vi "getExcitation.vi"(8 "error in (no error)":errorcluster, 11 "Inst.AH2500 in":refnum<class "Inst.AH2500.lvclass">) -> (0 "error out":errorcluster, 2 "Excitation (V)":dbl, 3 "Inst.AH2500 out":refnum<class "Inst.AH2500.lvclass">)   [LabVIEW 2019, in "Inst.AH2500.lvclass"]
uses:
  Inst.AH2500.lvclass
  C:/Program Files/National Instruments/LabVIEW 2019/user.lib/LevyLab/Instrument Framework/Instrument/Instrument.lvclass
  Typedefs/Inst.AH2500.Commands--Enum.ctl
  Typedefs/Inst.AH2500.getAll--Cluster.ctl
  991804cd-2d63-4689-a149-8f7b841441b7.vi/c179c0c8-4b72-489b-bcdd-bdfffdae94c9.vi
  991804cd-2d63-4689-a149-8f7b841441b7.vi/c179c0c8-4b72-489b-bcdd-bdfffdae94c9.vi/045b885c-8c33-4e8e-937d-f5afebc728a8.vi
  991804cd-2d63-4689-a149-8f7b841441b7.vi/c179c0c8-4b72-489b-bcdd-bdfffdae94c9.vi/f638782e-dab2-4f71-a606-cfbdff2ea2be.vi
  <vilib>/Utility/Data Type/Get Type Information.vi
  <vilib>/JDP Science/JSONtext/JSON text to Variant.vi
  <vilib>/JDP Science/JSONtext/LVClass Serializer/JSONtext LVClass Serializer.lvclass
  <userlib>/LevyLab/Instrument Framework/Instrument/Instrument.lvclass
  f3cb8313-5d80-4493-8332-6bf410390232.vi
  C:/Program Files/National Instruments/LabVIEW 2019/user.lib/LevyLab/Instrument Framework/Instrument Types/CBridge/Instrument.CBridge.lvclass
  C:/Program Files/National Instruments/LabVIEW 2019/vi.lib/JKI/JKI SMO/SMO/SMO.lvclass
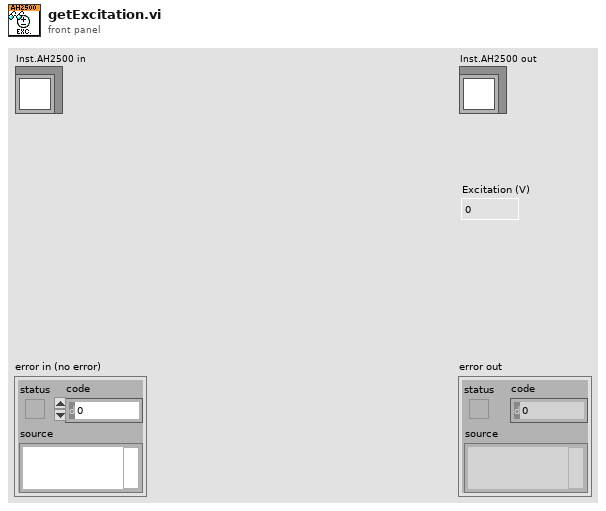
[diagram p1: front panel]
types:
  T1 = typedef "Inst.AH2500.lvclass/Inst.AH2500.getAll--Cluster.ctl" = cluster{"capacitance (pF)":dbl, "loss (nS)":dbl, "Vexc (V)":dbl}
  T2 = typedef "Inst.AH2500.lvclass/Inst.AH2500.Commands--Enum.ctl" = enum16{"getCapacitance", "getLoss", "getExcitation"}
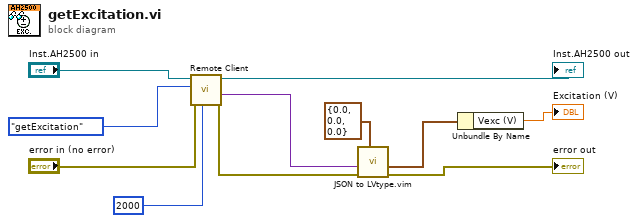
[diagram p0: block diagram]
diagram:
  n1 = call <userlib>:"Remote Client.vi"("timeout (ms) [500]"=2000 ("timeout (ms) test string"), "error in (no error)"="error in (no error)", "Command in"=Inst.AH2500.Commands--Enum."getExcitation" ("Commands"), "Instrument in"="Inst.AH2500 in") -> ("error out"=w7:errorcluster, "Data out"=w8:variant, "Instrument out"=→"Inst.AH2500 out":refnum<class "Inst.AH2500.lvclass">)  [unwired: 4 in, 1 out]
  n2 = call "JSON to LVtype.vim"("type"=T1 {"capacitance (pF)"=0.0, "loss (nS)"=0.0, "Vexc (V)"=0.0} ("getAll"), "error in (no error)"=w7, "JSON Data in"=w8) -> ("error out"=→"error out":errorcluster, "Data out"=w9:T1)  [unwired: 7 in]
  n3 = Unbundle By Name(w9) -> ("Vexc (V)"=→"Excitation (V)":dbl)
